vi "properties.get.vi"(8 "error in (no error)":errorcluster, 11 "asset in":refnum<class "asset.lvclass">) -> (0 "error out":errorcluster, 2 "nominal types.lvlib:properties.lvclass":refnum<class "properties.lvclass">, 3 "asset out":refnum<class "asset.lvclass">)   [LabVIEW 2020, in "asset.lvclass"]
uses:
  asset.lvclass
  nominal types/properties/properties.lvclass
  asset.lvclass/asset.ctl
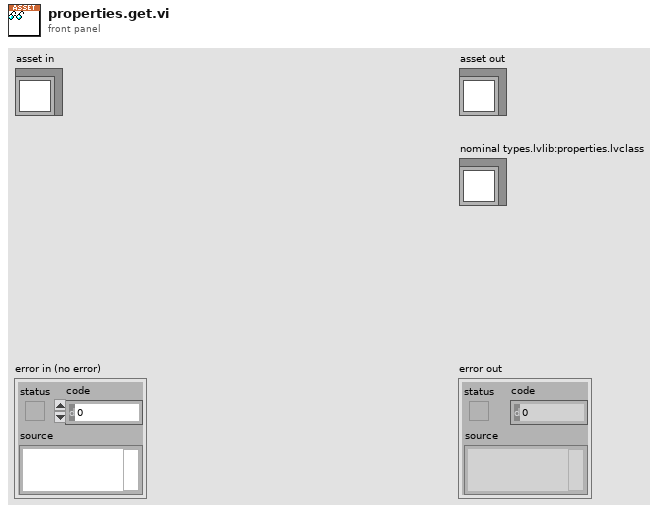
[diagram p1: front panel]
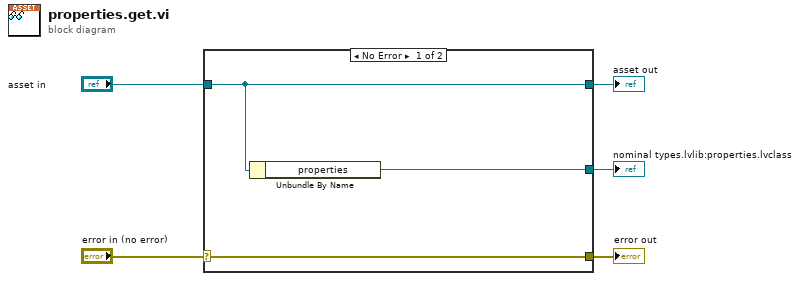
[diagram p0: block diagram]
diagram:
  n1 = case shown="No Error" "error in (no error)" {
    selector: "error in (no error)" -> [w8 w9]
    tunnel: [w8 w9] -> w4
    tunnel: [w7 w10] -> w2
    tunnel: "asset in" -> [w7 w10]
    tunnel: [w6 _] -> w1
    frame No Error {
      n2 = Unbundle By Name(w7) -> ("properties"=w6:refnum<class "properties.lvclass">)
    }
    frame Error {
    }
  }
  "error out" <- w4
  "asset out" <- w2
  "nominal types.lvlib:properties.lvclass" <- w1
